vi "电流.vi"(8 "error in":errorcluster, 11 "physical channels":tag="Dev1/ai4" caption="物理通道") -> (0 "error out":errorcluster)   [LabVIEW 2013]
uses:
  <vilib>/DAQmx/read.llb/DAQmx Read (Analog Wfm 1Chan NSamp).vi
  <vilib>/DAQmx/create/channels.llb/DAQmx Create Channel (AI-Voltage-Basic).vi
  <vilib>/DAQmx/configure/timing.llb/DAQmx Timing (Sample Clock).vi
  <vilib>/measure/madcrms.llb/Basic Averaged DC-RMS for 1 Chan.vi
  <vilib>/DAQmx/miscellaneous.llb/DAQmx Fill In Error Info.vi
  <vilib>/measure/NI_MAPro.lvlib
panel:
  in  "input terminal configuration 2":i32(ring)=-1 caption="输入接线端配置" items=["默认"=-1, "RSE"=10083, "NRSE"=10078, "差分"=10106, "伪差分"=12529]
  out "DC values":dbl[](array[numeric])=[5.536243745674683, 2.1639204614823164] caption="直流值" format="%.2p"
  in  "input terminal configuration":i32(ring)=10078 items=["default"=-1, "RSE"=10083, "NRSE"=10078, "Differential"=10106, "Pseudodifferential"=12529]
  out "电流":dbl=0.6945448692799161
  out "波形图表":waveform(dbl)(graph)={"t0"=timestamp(3479246323.546885 s since 1904-01-01), "dt"=9.999999999999972e-06, "Y"=array[100000 elements], "attributes"=variant("NI_ChannelName"=variant(string "Dev1/ai4"), "NI_UnitDescription"=variant(string "Volts"))}
  in  "布尔":bool
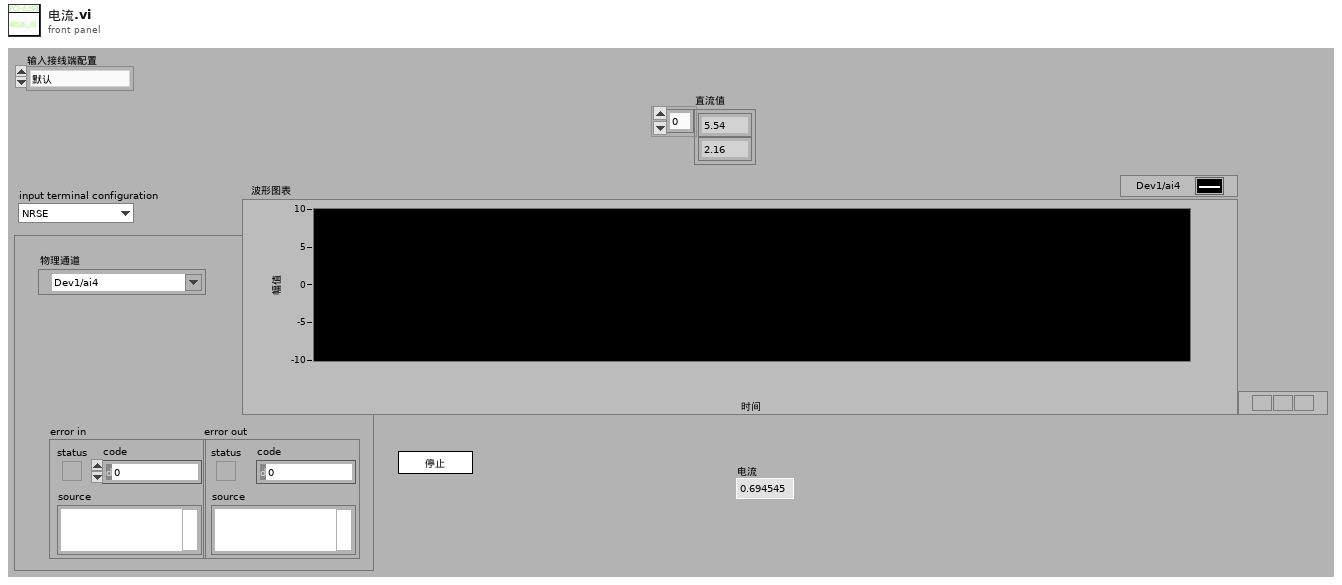
[diagram p1: front panel]
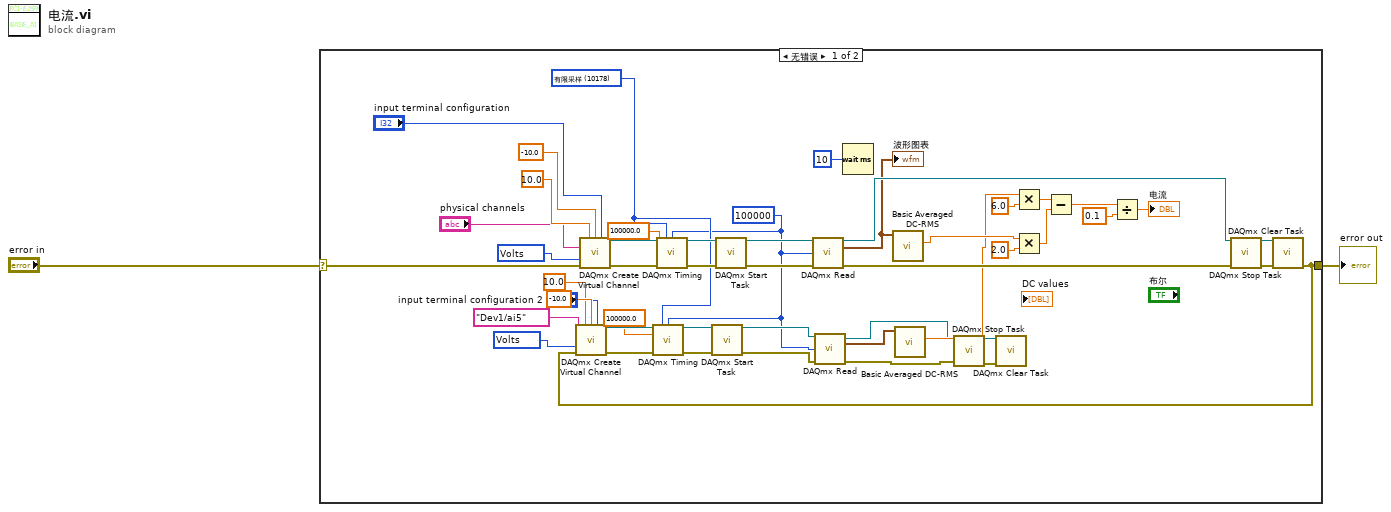
[diagram p0: block diagram]
diagram:
  n1 = case shown="无错误" "error in" {
    selector: "error in" -> [w43 w51]
    tunnel: [w9 w51] -> w2
    frame No Error {
      w4 = 100000 ("number of samples per channel")
      w30 = 10348 items=["Volts"=10348, "From Custom Scale"=10065] ("units")
      w26 = 10178 items=["有限采样"=10178, "连续采样"=10123, "硬件定时单点"=12522] ("sample mode")
      w48 = 10348 items=["Volts"=10348, "From Custom Scale"=10065] ("units")
      n2 = call-poly <vilib>:"DAQmx Create Virtual Channel.vi"("maximum value"=10.0, "minimum value"=-10.0, "input terminal configuration"="input terminal configuration", "physical channels"="physical channels", "units"=w48, "error in"=w43) -> ("task out"=w41:refnum<k21>, "error out"=w40:errorcluster)  [unwired: 8 in]
      n3 = call-poly <vilib>:"DAQmx Timing.vi"("task/channels in"=w41, "sample mode"=w26, "samples per channel"=w4, "rate"=100000.0, "error in"=w40) -> ("task out"=w39:refnum<k21>, "error out"=w38:errorcluster)  [unwired: 2 in, 7 out]
      n4 = call <vilib>:"DAQmx Start Task.vi"("task/channels in"=w39, "error in"=w38) -> ("task out"=w36:refnum<k21>, "error out"=w37:errorcluster)  [unwired: 12 in]
      n5 = call-poly <vilib>:"DAQmx Read.vi"("task/channels in"=w36, "number of samples per channel"=w4, "error in"=w37) -> ("task out"=w47:refnum<k21>, "data"=w21:waveform(dbl), "error out"=w46:errorcluster)  [unwired: 10 in]
      "波形图表" <- w21
      n6 = Wait (ms)(milliseconds to wait=u32 10 ("等待时间（毫秒）")) -> ()  [unwired: 1 out]
      n7 = call-poly <vilib>:"Basic Averaged DC-RMS.vi"("signal in"=w21) -> ("RMS value"=w12:dbl)  [unwired: 7 in, 3 out]
      n8 = Multiply(x=w12, y=2.0) -> (x*y=w15:dbl)
      n9 = call <vilib>:"DAQmx Stop Task.vi"("task/channels in"=w47, "error in"=w46) -> ("task out"=w50:refnum<k21>, "error out"=w49:errorcluster)  [unwired: 12 in]
      n10 = call <vilib>:"DAQmx Clear Task.vi"("task in"=w50, "error in"=w49) -> ("error out"=w9:errorcluster)  [unwired: 13 in]
      n11 = call-poly <vilib>:"DAQmx Create Virtual Channel.vi"("maximum value"=10.0, "minimum value"=-10.0, "input terminal configuration"="input terminal configuration 2", "physical channels"=tag "Dev1/ai5", "units"=w30, "error in"=w9) -> ("task out"=w31:refnum<k21>, "error out"=w32:errorcluster)  [unwired: 8 in]
      n12 = call-poly <vilib>:"DAQmx Timing.vi"("task/channels in"=w31, "sample mode"=w26, "samples per channel"=w4, "rate"=100000.0, "error in"=w32) -> ("task out"=w33:refnum<k21>, "error out"=w34:errorcluster)  [unwired: 2 in, 7 out]
      n13 = call <vilib>:"DAQmx Start Task.vi"("task/channels in"=w33, "error in"=w34) -> ("task out"=w27:refnum<k21>, "error out"=w10:errorcluster)  [unwired: 12 in]
      n14 = call-poly <vilib>:"DAQmx Read.vi"("task/channels in"=w27, "number of samples per channel"=w4, "error in"=w10) -> ("task out"=w7:refnum<k21>, "data"=w13:waveform(dbl), "error out"=w6:errorcluster)  [unwired: 10 in]
      n15 = call-poly <vilib>:"Basic Averaged DC-RMS.vi"("signal in"=w13) -> ("RMS value"=w11:dbl)  [unwired: 7 in, 3 out]
      n16 = call <vilib>:"DAQmx Stop Task.vi"("task/channels in"=w7, "error in"=w6) -> ("task out"=w5:refnum<k21>, "error out"=w8:errorcluster)  [unwired: 12 in]
      n17 = call <vilib>:"DAQmx Clear Task.vi"("task in"=w5, "error in"=w8) -> ()  [unwired: 13 in, 1 out]
      n18 = Multiply(x=w11, y=6.0) -> (x*y=w16:dbl)
      n19 = Subtract(x=w16, y=w15) -> (x-y=w14:dbl)
      n20 = Divide(x=w14, y=0.1) -> (x/y=→"电流":dbl)
    }
    frame Error {
    }
  }
  "error out" <- w2
